vi "Virtual Camera Get Temperature.vi"(8 "error in (no error)":errorcluster, 11 "Virtual Camera in":refnum<class "Virtual Camera.lvclass">) -> (0 "error out":errorcluster, 3 "Virtual Camera out":refnum<class "Virtual Camera.lvclass">)   [LabVIEW 2015]
uses:
  Virtual Camera.lvclass
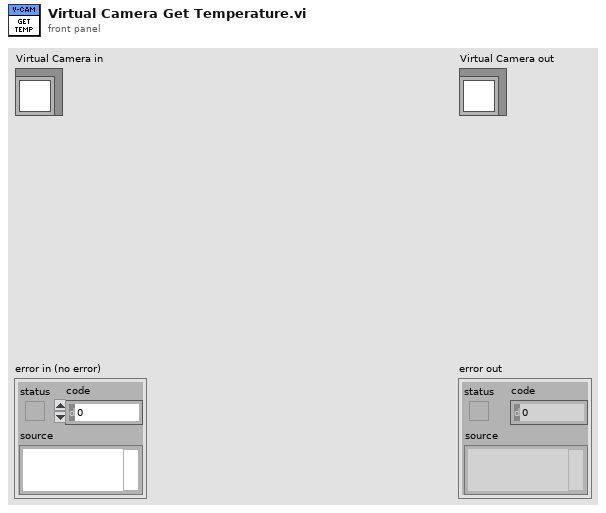
[diagram p1: front panel]
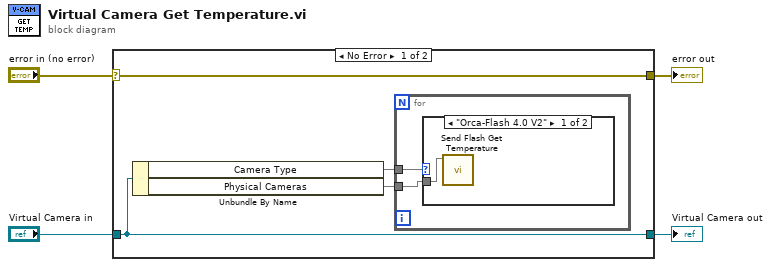
[diagram p0: block diagram]
diagram:
  n1 = case shown="No Error" "error in (no error)" {
    selector: "error in (no error)" -> [w8 w13]
    tunnel: [w8 w13] -> w3
    tunnel: [w7 w12] -> w1
    tunnel: "Virtual Camera in" -> [w7 w12]
    frame No Error {
      n2 = Unbundle By Name(w7) -> ("Camera Type"=w6, "Physical Cameras"=w5)
      n3 = for {
        tunnel: w6 -> [w10]
        tunnel: w5 -> [w9]
        n4 = case shown="\"Orca-Flash 4.0 V2\"" w10 {
          tunnel: w9 -> [w11 _]
          frame "Orca-Flash 4.0 V2" {
            n5 = call "Send Flash Get Temperature.vi"("Message Enqueuer"=w11) -> ()  [unwired: 9 in, 2 out]
          }
          frame Default {
          }
        }
      }
    }
    frame Error {
    }
  }
  "error out" <- w3
  "Virtual Camera out" <- w1
